vi "CarayaCLIExecutionEngine.vi"() -> ()   [LabVIEW 2013]
uses:
  <vilib>/Wiresmith Technology/G CLI/CLI Class/CLI.lvclass
  <vilib>/addons/_JKI Toolkits/Caraya/Caraya.lvlib
panel:
  out "error out":errorcluster
  out "source folder":path
  out "report filename":string
  out "Application:Command Line Arguments":string[](array[string])
  out "recursive":bool
  out "verbose":bool
  out "Interactive":bool
  out "output path":path
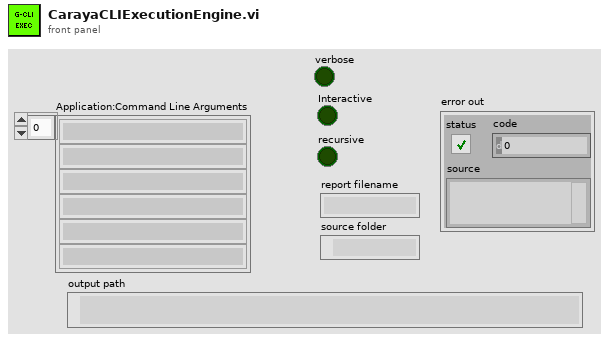
[diagram p1: front panel]
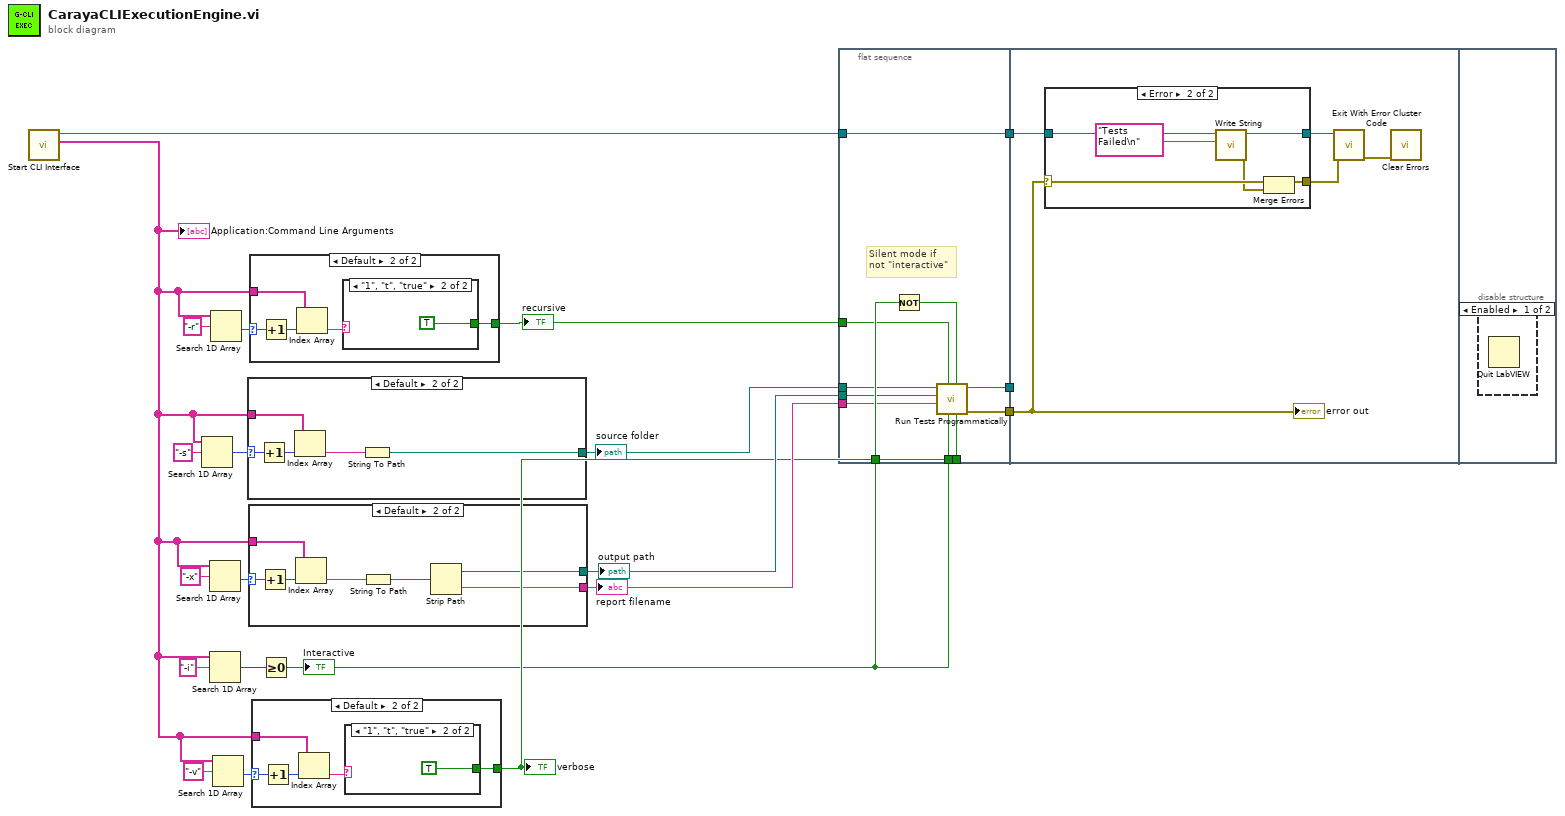
[diagram p0: block diagram]
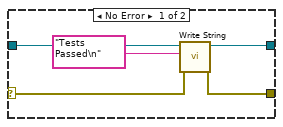
[diagram p2: hidden frame]
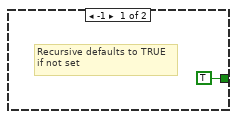
[diagram p6: hidden frame]
diagram:
  n1 = call <vilib>:"Start CLI Interface.vi"() -> ("Custom Parameters"=w5:string[], "CLI out"=w4:refnum<class "CLI.lvclass">)  [unwired: 8 in, 2 out]
  "Application:Command Line Arguments" <- w5
  n2 = Search 1D Array(1D array=w5, element="-s") -> (index of element=w12:i32)  [unwired: 1 in]
  n3 = Search 1D Array(1D array=w5, element="-x") -> (index of element=w14:i32)  [unwired: 1 in]
  n4 = Search 1D Array(1D array=w5, element="-i") -> (index of element=w20:i32)  [unwired: 1 in]
  n5 = Search 1D Array(1D array=w5, element="-r") -> (index of element=w17:i32)  [unwired: 1 in]
  n6 = Search 1D Array(1D array=w5, element="-v") -> (index of element=w18:i32)  [unwired: 1 in]
  n7 = case shown="Default" w12 {
    selector: w12 -> [_ w25]
    tunnel: w5 -> [_ w24]
    tunnel: [_ w22] -> w11
    frame -1 {
    }
    frame Default {
      n8 = Increment(x=w25) -> (x+1=w26:i32)
      n9 = Index Array(array=w24, index=w26) -> (element=w23:string)
      n10 = String To Path(string=w23) -> (path=w22:path)
    }
  }
  "source folder" <- w11
  n11 = case shown="Default" w14 {
    selector: w14 -> [_ w32]
    tunnel: w5 -> [_ w31]
    tunnel: [_ w28] -> w10
    tunnel: [_ w27] -> w9
    frame -1 {
    }
    frame Default {
      n12 = Increment(x=w32) -> (x+1=w33:i32)
      n13 = Index Array(array=w31, index=w33) -> (element=w30:string)
      n14 = String To Path(string=w30) -> (path=w29:path)
      n15 = Strip Path(path=w29) -> (stripped path=w28:path, name=w27:string)
    }
  }
  "output path" <- w10
  "report filename" <- w9
  n16 = case shown="Default" w17 {
    selector: w17 -> [_ w36]
    tunnel: [TRUE w37] -> w8
    tunnel: w5 -> [_ w35]
    frame -1 {
      # "Recursive defaults to TRUE\nif not set"
    }
    frame Default {
      n17 = Increment(x=w36) -> (x+1=w39:i32)
      n18 = Index Array(array=w35, index=w39) -> (element=w38:string)
      n19 = case shown="\"1\", \"t\", \"true\"" w38 {
        tunnel: [_ TRUE] -> w37
        frame Default {
        }
        frame "1", "t", "true" {
        }
      }
    }
  }
  "recursive" <- w8
  n20 = case shown="Default" w18 {
    selector: w18 -> [_ w42]
    tunnel: [_ w43] -> w7
    tunnel: w5 -> [_ w41]
    frame -1 {
      # "Verosity defaults to False\nif not set"
    }
    frame Default {
      n21 = Increment(x=w42) -> (x+1=w45:i32)
      n22 = Index Array(array=w41, index=w45) -> (element=w44:string)
      n23 = case shown="\"1\", \"t\", \"true\"" w44 {
        tunnel: [_ TRUE] -> w43
        frame Default {
        }
        frame "1", "t", "true" {
        }
      }
    }
  }
  "verbose" <- w7
  n24 = Greater Or Equal To 0?(x=w20) -> (x >= 0?=w6:bool)
  "Interactive" <- w6
  n25 = flat-sequence {
    tunnel: w11 -> [w55]
    tunnel: w10 -> [w52]
    tunnel: w9 -> [w51]
    tunnel: w8 -> [w54]
    tunnel: w6 -> [w50]
    tunnel: w7 -> [w49]
    tunnel: w6 -> [w57]
    tunnel: w4 -> [w56]
    tunnel: [w56] -> w3
    tunnel: [w48] -> w2
    tunnel: [w47] -> w1
    tunnel: w3 -> [w61]
    tunnel: w2 -> [w59]
    tunnel: w1 -> [_]
    frame #0 {
      # "Silent mode if\nnot \"interactive\""
      n26 = Not(x=w57) -> (.not. x?=w53:bool)
      n27 = call <vilib>:"Run Tests Programmatically.vi"("Verbose"=w49, "Silent"=w53, "Interactive"=w50, "Inspect Recursively"=w54, "Report name"=w51, "Output Folder"=w52, "Source Folder"=w55) -> ("error out"=w48:errorcluster, "Test Runner"=w47:refnum<class "Test Runner.lvclass">)  [unwired: 3 in]
    }
    frame #1 {
      n28 = case shown="Error" w59 {
        selector: w59 -> [w64 w70]
        tunnel: w61 -> [w67 w73]
        tunnel: [w66 w72] -> w60
        tunnel: [w63 w68] -> w58
        frame No Error {
          n29 = call <vilib>:"Write String.vi"("error in (no error)"=w64, "Text to Write"="Tests Passed\n", "CLI in"=w67) -> ("error out"=w63:errorcluster, "CLI out"=w66:refnum<class "CLI.lvclass">)  [unwired: 7 in]
        }
        frame Error {
          n30 = call <vilib>:"Write String.vi"("Text to Write"="Tests Failed\n", "CLI in"=w73) -> ("error out"=w69:errorcluster, "CLI out"=w72:refnum<class "CLI.lvclass">)  [unwired: 8 in]
          n31 = Merge Errors(w70, w69) -> (w68:errorcluster)
        }
      }
      n32 = call <vilib>:"Exit With Error Cluster Code.vi"("error in (no error)"=w58, "CLI in"=w60) -> ("error out"=w62:errorcluster)  [unwired: 9 in]
      n33 = call <vilib>:"Clear Errors.vi"("error in (no error)"=w62) -> ()  [unwired: 6 in, 1 out]
      "error out" <- w59
    }
    frame #2 {
      n34 = disable-structure shown="Enabled" {
        frame Enabled {
          n35 = Quit LabVIEW() -> ()  [unwired: 1 in]
        }
        frame Disabled {
        }
      }
    }
  }
